vi "sendCloseEvent.vi"(8 "error in (no error)":errorcluster, 11 "ScriptEvent in":refnum<class "ScriptEvent.lvclass">) -> (0 "error out":errorcluster, 3 "ScriptEvent out":refnum<class "ScriptEvent.lvclass">)   [LabVIEW 2011, in "Events.lvlib" / "ScriptEvent.lvclass"]
uses:
  ScriptEvent.lvclass
  ScriptEvent.lvclass/ScriptEvent.ctl
  Event.lvclass
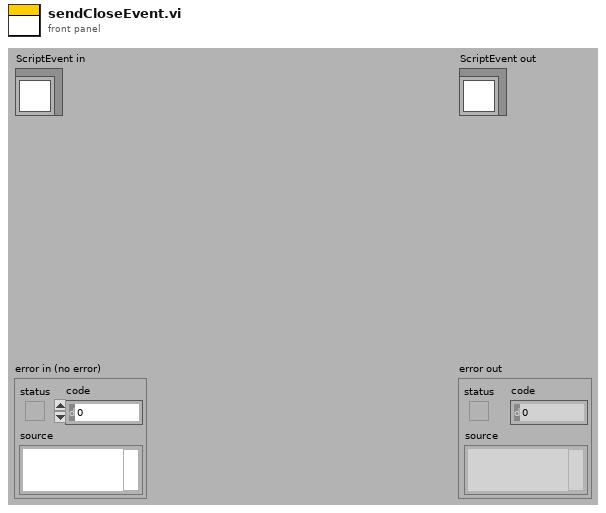
[diagram p1: front panel]
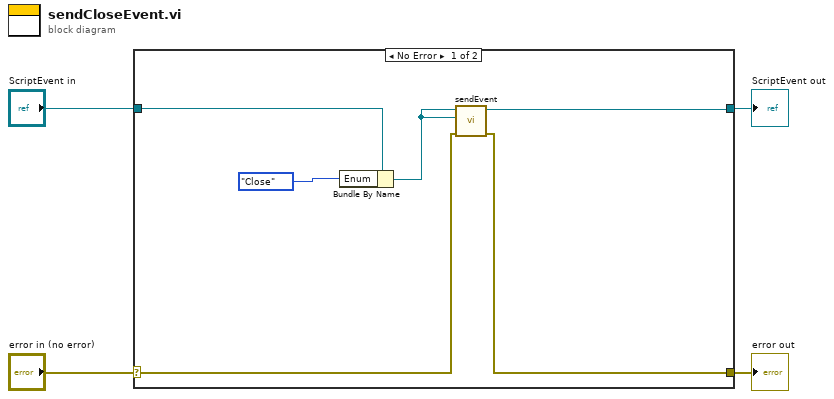
[diagram p0: block diagram]
diagram:
  n1 = case shown="No Error" "error in (no error)" {
    selector: "error in (no error)" -> [w6 w12]
    tunnel: [w5 w12] -> w3
    tunnel: [w8 w11] -> w1
    tunnel: "ScriptEvent in" -> [w9 w11]
    frame No Error {
      n2 = Bundle By Name(cluster=w9, "Enum"=enum16{"Open", "Save", "Close"}."Close") -> (w7:refnum<class "ScriptEvent.lvclass">)
      n3 = call "sendEvent.vi"("error in (no error)"=w6, "data"=w7, "Event in"=w7) -> ("error out"=w5:errorcluster, "Event out"=w8:refnum<class "ScriptEvent.lvclass">)  [unwired: 7 in]
    }
    frame Error {
    }
  }
  "error out" <- w3
  "ScriptEvent out" <- w1
